vi "Joints Example.vi"() -> ()   [LabVIEW 2016]
doc: "Example VI: reads in and writes to Baxter's joint states"
uses:
  ROS/Code/JointPositions.ctl
  ROS/Code/Slider.ctl
panel:
  in  "Bring Arms In":bool
  in  "Reset to Zero":bool
  in  "Joint Positions":T1 {"left_w2" scale=-180.0..180.0; "left_w1" scale=-180.0..180.0; "left_w0" scale=-180.0..180.0; "left_e1" scale=-180.0..180.0; "left_e0" scale=-180.0..180.0; "left_s1" scale=-180.0..180.0; "left_s0" scale=-180.0..180.0; "right_s1" scale=-180.0..180.0; "right_s0" scale=-180.0..180.0; "right_w2" scale=-180.0..180.0; "right_e1" scale=-180.0..180.0; "right_e0" scale=-180.0..180.0; "right_w0" scale=-180.0..180.0; "right_w1" scale=-180.0..180.0}
  in  "stop":bool
  # "Control Baxter's Arms using the supplied Position Controller"
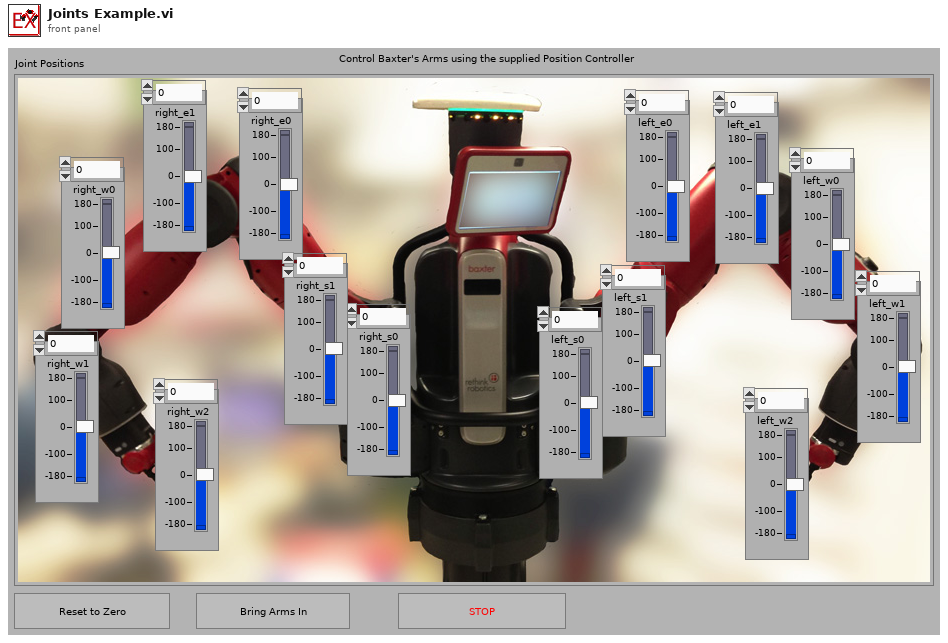
[diagram p1: front panel]
types:
  T1 = typedef "JointPositions.ctl" = cluster{"left_e0":T2, "left_e1":T2, "left_s0":T2, "left_s1":T2, "left_w0":T2, "left_w1":T2, "left_w2":T2, "right_e0":T2, "right_e1":T2, "right_s0":T2, "right_s1":T2, "right_w0":T2, "right_w1":T2, "right_w2":T2}
  T2 = typedef "Slider.ctl" = dbl
  T3 = cluster{"Joint Name":string, "Position":dbl, "Velocity":dbl, "Effort":dbl}[]
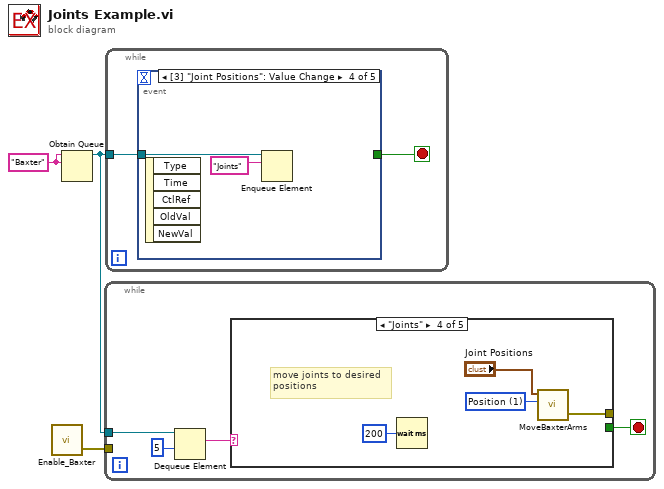
[diagram p0: block diagram]
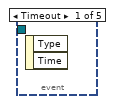
[diagram p2: hidden frame]
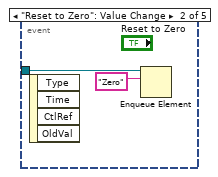
[diagram p3: hidden frame]
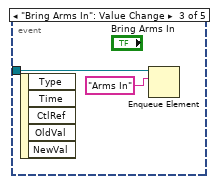
[diagram p4: hidden frame]
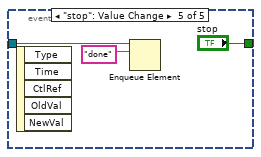
[diagram p5: hidden frame]
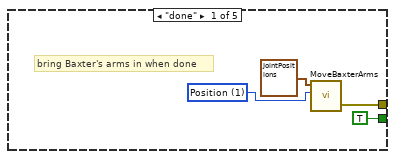
[diagram p6: hidden frame]
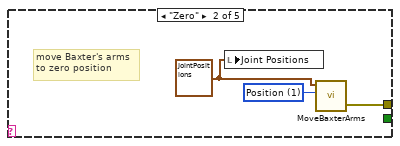
[diagram p7: hidden frame]
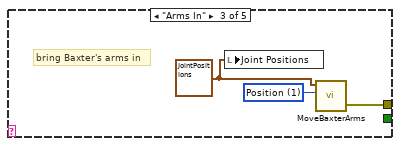
[diagram p8: hidden frame]
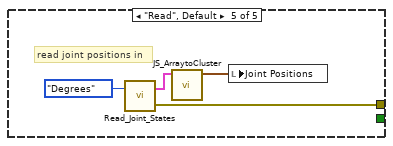
[diagram p9: hidden frame]
diagram:
  w2 = "Baxter" ("name (unnamed)")
  n1 = call "Enable_Baxter.vi"() -> ("error out"=w1:errorcluster)  [unwired: 4 in]
  n2 = Obtain Queue(name (unnamed)=w2, element data type=w2) -> (queue out=w3:refnum<queue>)  [unwired: 3 in, 2 out]
  n3 = while {
    tunnel: w3 -> [w7]
    tunnel: w1 -> [_]
    stop <- w5 stop-if-true
    n4 = Dequeue Element(queue=w7, timeout in ms (-1)=5) -> (element=w6:string)  [unwired: 1 in, 3 out]
    n5 = case shown="\"Joints\"" w6 {
      tunnel: [TRUE ("stop") _ _ _ _] -> w5
      tunnel: [w8 w12 w15 w20 w23] -> _
      frame "done" {
        w10 = u8 1 items=["Position"=1, "Velocity"=2, "Effort"=3] ("Mode")
        # "bring Baxter's arms in when done"
        n6 = call "MoveBaxterArms.vi"("Parameters"=T1 {"left_e0"=0.0, "left_e1"=90.0, "left_s0"=-30.0, "left_s1"=0.0, "left_w0"=0.0, "left_w1"=0.0, "left_w2"=0.0, "right_e0"=0.0, "right_e1"=90.0, "right_s0"=30.0, "right_s1"=0.0, "right_w0"=0.0, "right_w1"=0.0, "right_w2"=0.0} ("Joint Positions 2"), "Mode"=w10) -> ("error out"=w8:errorcluster)  [unwired: 4 in]
      }
      frame "Zero" {
        w13 = u8 1 items=["Position"=1, "Velocity"=2, "Effort"=3] ("Mode")
        w14 = T1 {"left_e0"=0.0, "left_e1"=0.0, "left_s0"=0.0, "left_s1"=0.0, "left_w0"=0.0, "left_w1"=0.0, "left_w2"=0.0, "right_e0"=0.0, "right_e1"=0.0, "right_s0"=0.0, "right_s1"=0.0, "right_w0"=0.0, "right_w1"=0.0, "right_w2"=0.0} ("Joint Positions 2")
        # "move Baxter's arms\nto zero position"
        n7 = local write "Joint Positions"(w14) -> ()
        n8 = call "MoveBaxterArms.vi"("Parameters"=w14, "Mode"=w13) -> ("error out"=w12:errorcluster)  [unwired: 4 in]
      }
      frame "Arms In" {
        w16 = u8 1 items=["Position"=1, "Velocity"=2, "Effort"=3] ("Mode")
        w17 = T1 {"left_e0"=0.0, "left_e1"=90.0, "left_s0"=-30.0, "left_s1"=0.0, "left_w0"=0.0, "left_w1"=0.0, "left_w2"=0.0, "right_e0"=0.0, "right_e1"=90.0, "right_s0"=30.0, "right_s1"=0.0, "right_w0"=0.0, "right_w1"=0.0, "right_w2"=0.0} ("Joint Positions 2")
        # "bring Baxter's arms in"
        n9 = local write "Joint Positions"(w17) -> ()
        n10 = call "MoveBaxterArms.vi"("Parameters"=w17, "Mode"=w16) -> ("error out"=w15:errorcluster)  [unwired: 4 in]
      }
      frame "Joints" {
        w21 = u8 1 items=["Position"=1, "Velocity"=2, "Effort"=3] ("Mode")
        # "move joints to desired\npositions"
        n11 = Wait (ms)(milliseconds to wait=u32 200) -> ()  [unwired: 1 out]
        n12 = call "MoveBaxterArms.vi"("Parameters"="Joint Positions", "Mode"=w21) -> ("error out"=w20:errorcluster)  [unwired: 4 in]
      }
      frame "Read", Default {
        # "read joint positions in"
        n13 = call "Read_Joint_States.vi"("Units (deg)"=enum16{"Radians", "Degrees"}."Degrees") -> ("error out"=w23:errorcluster, "Joint States"=w25:T3)  [unwired: 2 in]
        n14 = call "JS_ArraytoCluster.vi"("Joint States"=w25) -> ("Joint Positions 2"=w22:T1)  [unwired: 10 in]
        n15 = local write "Joint Positions"(w22) -> ()
      }
    }
  }
  n16 = while {
    tunnel: w3 -> [w26]
    stop <- w27 stop-if-true
    n17 = event shown="[3] \"Joint Positions\": Value Change" {
      selector: _ -> [_ _ _ _ _]
      dyn-events: _ -> [_ _ _ _ _]
      timeout: _ -> [_ _ _ _ _]
      tunnel: [_ _ _ _ "stop"] -> w27
      tunnel: w26 -> [_ w28 w30 w32 w35]
      event Timeout {
        n18 = event-data() -> ()  [unwired: 1 in, 2 out]
      }
      event "Reset to Zero": Value Change {
        n19 = event-data() -> ()  [unwired: 1 in, 4 out]
        n20 = Enqueue Element(queue=w28, element="Zero") -> ()  [unwired: 2 in, 3 out]
      }
      event "Bring Arms In": Value Change {
        n21 = event-data() -> ()  [unwired: 1 in, 5 out]
        n22 = Enqueue Element(queue=w30, element="Arms In") -> ()  [unwired: 2 in, 3 out]
      }
      event Value Change {
        n23 = event-data() -> ()  [unwired: 1 in, 5 out]
        n24 = Enqueue Element(queue=w32, element="Joints") -> ()  [unwired: 2 in, 3 out]
      }
      event "stop": Value Change {
        n25 = event-data() -> ()  [unwired: 1 in, 5 out]
        n26 = Enqueue Element(queue=w35, element="done") -> ()  [unwired: 2 in, 3 out]
      }
    }
  }
